vi "GetHelp.vi"(0 "XRef":T18, 1 "Point":T17, 2 "State In":T13 {"BlockNodeState"."Draw Style" items=["FunctionBlock", "ExpressVI", "Variable", "Elemental I/O", "32x32 Icon", "FunctionBlockCompact"]; "BlockNodeState"."Terminal Data"."Terminal Flags" format="%.0b"}) -> (14 "Standard Help Info":T12, 15 "Detailed Help Info":T9, 16 "Subitem Help Info":T4, 17 "Use Detailed Help?":T3, 18 "Use Subitem Help?":T3)   [LabVIEW 2017, in "NI_Robotics_Create Steering Frame.xnode"]
doc: "Generates a wheeled steering frame that you design in an interactive dialog box. You can choose from pre-defined steering frame designs or create a custom frame design."
uses:
  <vilib>/robotics/Steering/Create Steering Frame/NI_Robotics_Create Steering Frame.xnode
  <vilib>/XNodeSupport/XNodeXNodeRef.ctl
  <vilib>/XNodeSupport/XNodePoint.ctl
  <vilib>/XNodeSupport/XNodeInt.ctl
  <vilib>/robotics/Steering/Create Steering Frame/State.ctl
  <vilib>/BlockNodeSupport/BlockNodeState.ctl
  <vilib>/BlockNodeSupport/TerminalData.ctl
  <vilib>/picture/picture.llb/imagedata.ctl
  <vilib>/XNodeSupport/XNodeStandardHelpInfo.ctl
  <vilib>/XNodeSupport/XNodeString.ctl
  <vilib>/XNodeSupport/XNodePath.ctl
  <vilib>/XNodeSupport/XNodeDetailedHelpInfo.ctl
  <vilib>/XNodeSupport/XNodeImage.ctl
  <vilib>/XNodeSupport/XNodeRect32.ctl
  <vilib>/XNodeSupport/XNodeTerms.ctl
  <vilib>/XNodeSupport/XNodeTerm.ctl
  <vilib>/XNodeSupport/XNodeVariant.ctl
  <vilib>/XNodeSupport/XNodeBool.ctl
  <vilib>/XNodeSupport/XNodeSubitemHelpInfo.ctl
  <vilib>/XNodeSupport/NI_XNodeSupport.lvlib
panel:
  in  "Path":T1=path "<helpdir>/lvrobovi.chm"
  in  "Tag":T2="config_steering_frame.html"
  in  "Description":T2="Generates a wheeled steering frame that you design in an interactive dialog box. You can choose from pre-defined steering frame designs or create a custom frame design."
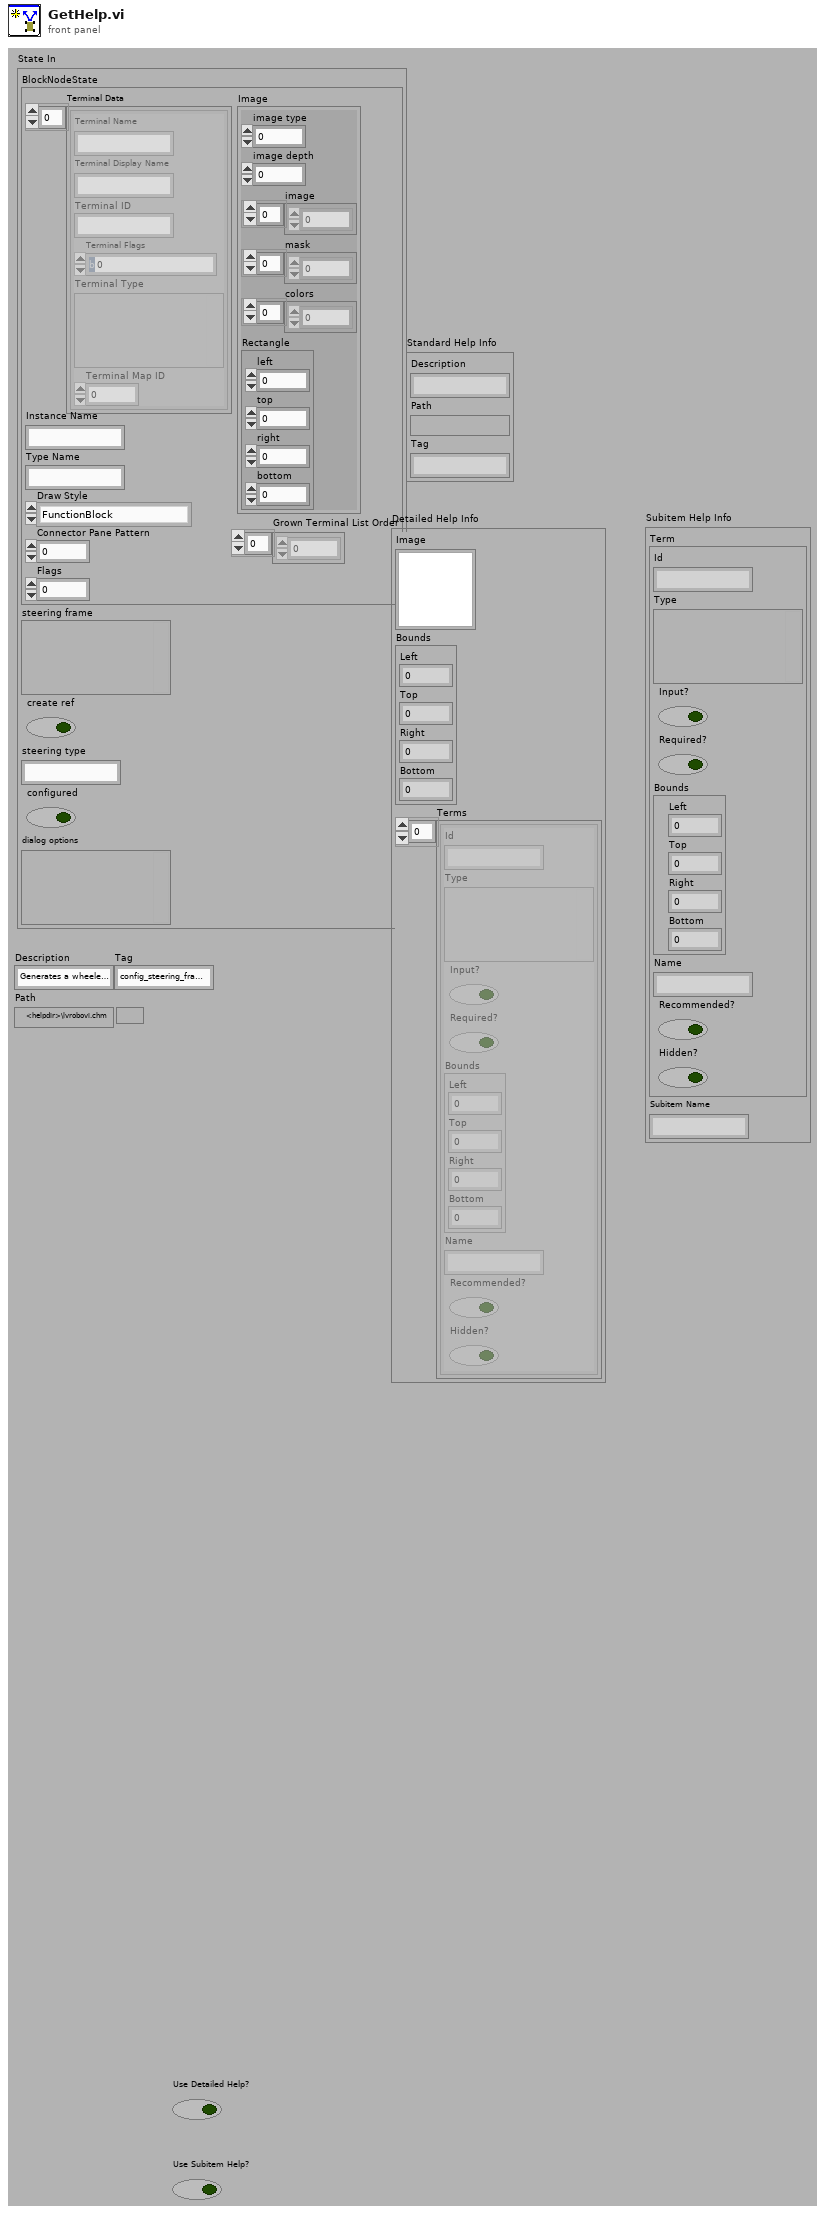
[diagram p1: front panel]
types:
  T1 = typedef "NI_XNodeSupport.lvlib/XNodePath.ctl" = path
  T2 = typedef "NI_XNodeSupport.lvlib/XNodeString.ctl" = string
  T3 = typedef "NI_XNodeSupport.lvlib/XNodeBool.ctl" = bool
  T4 = typedef "NI_XNodeSupport.lvlib/XNodeSubitemHelpInfo.ctl" = cluster{"Term":T5, "Subitem Name":T2}
  T5 = typedef "NI_XNodeSupport.lvlib/XNodeTerm.ctl" = cluster{"Id":T2, "Type":T6, "Input?":T3, "Required?":T3, "Bounds":T7, "Name":T2, "Recommended?":T3, "Hidden?":T3}
  T6 = typedef "NI_XNodeSupport.lvlib/XNodeVariant.ctl" = variant
  T7 = typedef "NI_XNodeSupport.lvlib/XNodeRect32.ctl" = cluster{"Left":T8, "Top":T8, "Right":T8, "Bottom":T8}
  T8 = typedef "NI_XNodeSupport.lvlib/XNodeInt.ctl" = i32
  T9 = typedef "NI_XNodeSupport.lvlib/XNodeDetailedHelpInfo.ctl" = cluster{"Image":T10, "Bounds":T7, "Terms":T11}
  T10 = typedef "NI_XNodeSupport.lvlib/XNodeImage.ctl" = picture
  T11 = typedef "NI_XNodeSupport.lvlib/XNodeTerms.ctl" = T5[]
  T12 = typedef "NI_XNodeSupport.lvlib/XNodeStandardHelpInfo.ctl" = cluster{"Description":T2, "Path":T1, "Tag":T2}
  T13 = typedef "NI_Robotics_Create Steering Frame.xnode/State.ctl" = cluster{"BlockNodeState":T14, "steering frame":variant, "create ref":bool, "steering type":string, "configured":bool, "dialog options":variant}
  T14 = typedef "BlockNodeState.ctl" = cluster{"Terminal Data":T15[], "Instance Name":string, "Type Name":string, "Draw Style":i32, "Connector Pane Pattern":i32, "Flags":i32, "Grown Terminal List Order":i32[], "Image":T16}
  T15 = typedef "TerminalData.ctl" = cluster{"Terminal Name":string, "Terminal Display Name":string, "Terminal ID":string, "Terminal Flags":i32, "Terminal Type":variant, "Terminal Map ID":i32}
  T16 = typedef "imagedata.ctl" = cluster{"image type":i32, "image depth":i32, "image":u8[], "mask":u8[], "colors":u32[], "Rectangle":cluster{"left":i16, "top":i16, "right":i16, "bottom":i16}}
  T17 = typedef "NI_XNodeSupport.lvlib/XNodePoint.ctl" = cluster{"H":T8, "V":T8}
  T18 = typedef "NI_XNodeSupport.lvlib/XNodeXNodeRef.ctl" = refnum<vi>
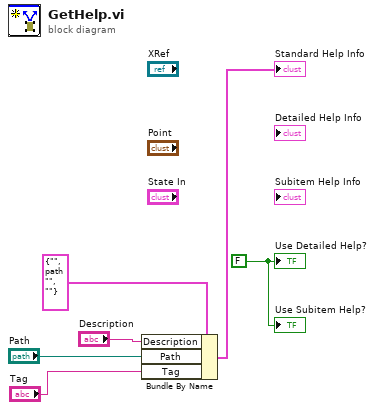
[diagram p0: block diagram]
diagram:
  w6 = T3 FALSE ("Use Detailed Help?")
  n1 = Bundle By Name(cluster=T12 {"Description"="", "Path"=path "", "Tag"=""} ("Standard Help Info"), "Description"="Description", "Path"="Path", "Tag"="Tag") -> (→"Standard Help Info":T12)
  "Use Detailed Help?" <- w6
  "Use Subitem Help?" <- w6
